vi "Get Resource Names By Type.vi"(8 "error in (no error)":errorcluster, 9 "Data Type":variant, 10 "Resource Type":T2(ring), 11 "Resource Info In":T1[](array[typedef])) -> (0 "error out":errorcluster, 2 "Resource Names":string[](array[string]), 3 "Resource Info Out (dup)":T1[](array[typedef]))   [LabVIEW 2017, in "NI_VDM_FPGA_Basics.lvlib"]
uses:
  <vilib>/NI/LVFPGA Adv Session Resources/ResourceInfo.ctl
  <vilib>/visionFPGA/NI_VDM_FPGA_Basics.lvlib
  <vilib>/NI/LVFPGA Adv Session Resources/LVFPGAAdvSessionResources.lvlib
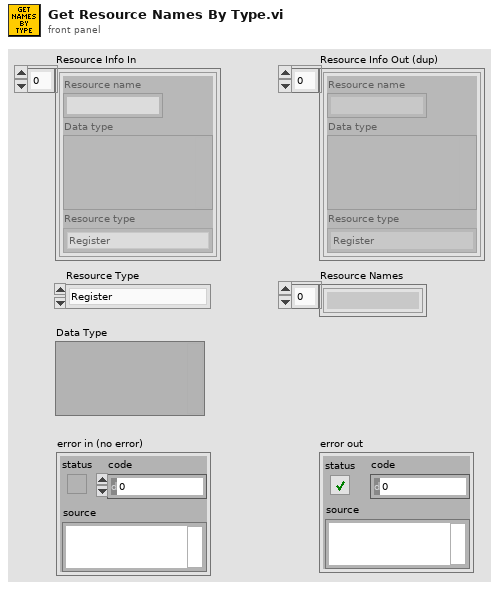
[diagram p1: front panel]
types:
  T1 = typedef "LVFPGAAdvSessionResources.lvlib/ResourceInfo.ctl" = cluster{"Resource name":string, "Data type":variant, "Resource type":enum16{"Register", "Host To Target FIFO", "Target To Host FIFO"}}
  T2 = enum16{"Register", "Host To Target FIFO", "Target To Host FIFO"}
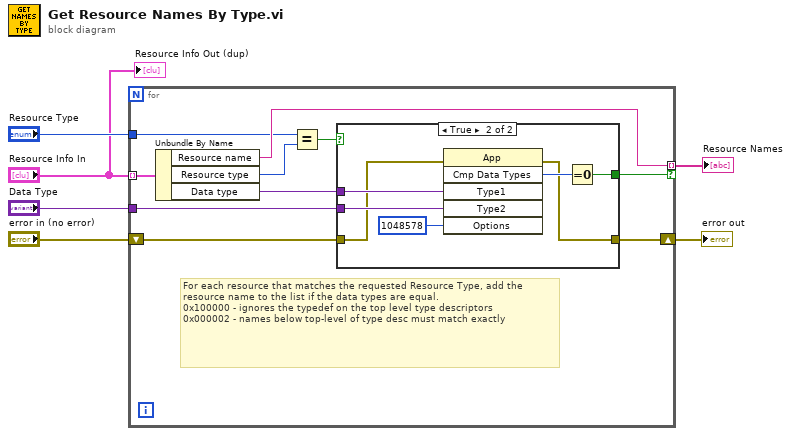
[diagram p0: block diagram]
diagram:
  n1 = for {
    tunnel: "Resource Info In" -> [w15] mode=indexing
    tunnel: [w14] -> w5 mode=indexing if=w10
    tunnel: "Data Type" -> [w13]
    shift-right: [w11] -> w6
    shift-left: "error in (no error)" -> [w12]
    tunnel: "Resource Type" -> [w9]
    # "For each resource that matches the requested Resource Type, add the resource name to the list if the data types are equal.\n0x100000 - ignores the typedef on the top level type descriptors\n0x000002 - names below top-level of type desc must match exactly"
    n2 = Unbundle By Name(w15) -> ("Resource name"=w14:string, "Resource type"=w8:T2, "Data type"=w16:variant)
    n3 = Equal?(x=w9, y=w8) -> (x = y?=w7:bool)
    n4 = case shown="True" w7 {
      tunnel: w16 -> [_ w23]
      tunnel: [_ w18] -> w10
      tunnel: w13 -> [_ w22]
      tunnel: w12 -> [w17 w21]
      tunnel: [w17 w19] -> w11
      frame False {
      }
      frame True {
        n5 = invoke class="App" method="Cmp Data Types"(error in=w21, "Type1"=w23, "Type2"=w22, "Options"=1048578) -> (error out=w19:errorcluster, "Compare Data Types"=w24:i32)  [unwired: 2 in, 4 out]
        n6 = Equal To 0?(x=w24) -> (x = 0?=w18:bool)
      }
    }
  }
  "error out" <- w6
  "Resource Names" <- w5
  "Resource Info Out (dup)" <- "Resource Info In"
